vi "读取状态输出.vi"(8 "error in (no error)":errorcluster caption="错误输入（无错误）", 11 "http client输入":refnum<class "http client.lvclass">) -> (0 "error out":errorcluster caption="错误输出", 2 "状态输出":refnum<notifier>, 3 "http client输出":refnum<class "http client.lvclass">)   [LabVIEW 2022 SP3, in "update.lvlib" / "http client.lvclass"]
uses:
  http client.lvclass
  http client.lvclass/http client.ctl
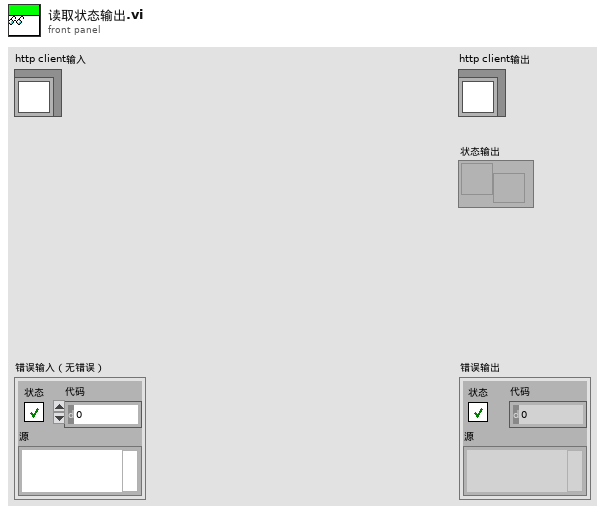
[diagram p1: front panel]
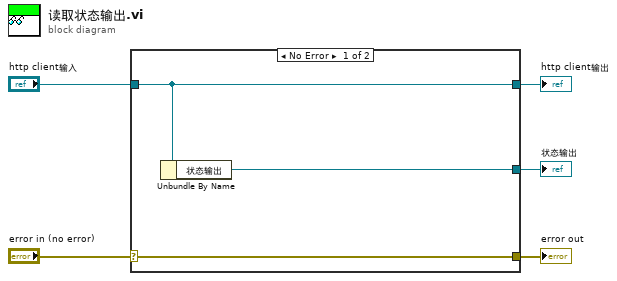
[diagram p0: block diagram]
diagram:
  n1 = case shown="No Error" "error in (no error)" {
    selector: "error in (no error)" -> [w8 w9]
    tunnel: [w8 w9] -> w4
    tunnel: [w7 w10] -> w2
    tunnel: "http client输入" -> [w7 w10]
    tunnel: [w6 _] -> w1
    frame No Error {
      n2 = Unbundle By Name(w7) -> ("状态输出"=w6:refnum<notifier>)
    }
    frame Error {
    }
  }
  "error out" <- w4
  "http client输出" <- w2
  "状态输出" <- w1
